vi "BRig_dataExp_init.vi"() -> (3 "output_dataExp":u16[](array[numeric]))   [LabVIEW 2014]
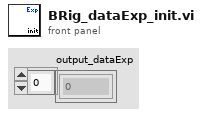
[diagram p1: front panel]
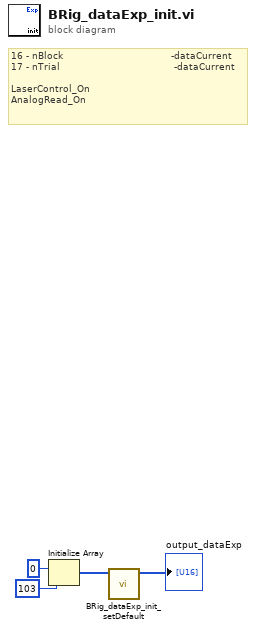
[diagram p0: block diagram]
diagram:
  # "16 - nBlock                                    -dataCurrent\n17 - nTrial                                      -dataCurrent\n\nLaserControl_On\nAnalogRead_On"
  n1 = Initialize Array(u16 0 ("element"), 103 ("dimension size")) -> (w2:u16[])
  n2 = call "BRig_dataExp_init_setDefault.vi"("input_dataExp"=w2) -> ("output_dataExp"=→"output_dataExp":u16[])  [unwired: 10 in]
